vi "StringRight.vi"(2 "#chars":i32=2, 3 "input string":string) -> (1 "output string":string)   [LabVIEW 2024]
doc: "Extracts the righmost n characters from string"
panel:
  # "Extracts the righmost n characters from string.\nAPR 2/23/2000"
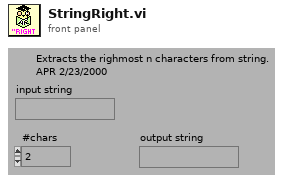
[diagram p1: front panel]
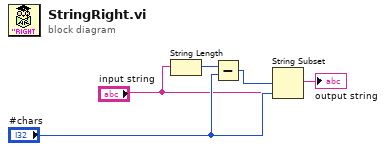
[diagram p0: block diagram]
diagram:
  n1 = String Length(string="input string") -> (length=w5:i32)
  n2 = Subtract(x=w5, y="#chars") -> (x-y=w3:i32)
  n3 = String Subset(string="input string", offset (0)=w3, length (rest)="#chars") -> (substring=→"output string":string)
